vi "AppendDBLtoComments.vi"(9 "Numeric":dbl, 10 "Label":string, 11 "Comments in":string) -> (3 "Comments out":string)   [LabVIEW 2016, in "SweepControl.lvclass"]
uses:
  SweepControl.lvclass
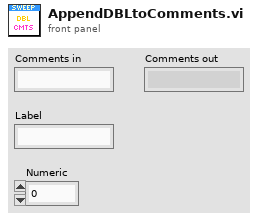
[diagram p1: front panel]
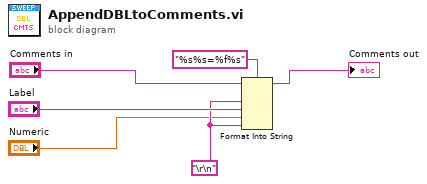
[diagram p0: block diagram]
diagram:
  w5 = "\r\n"
  n1 = Format Into String(format string="%s%s=%f%s", initial string="Comments in", w5, "Label", "Numeric", w5) -> (resulting string=→"Comments out":string)  [unwired: 1 in, 1 out]
